vi "PortsArrayHandler.vi"(2 "Input":u8[](array[numeric]), 3 "Init Input":u8[](array[numeric]), 4 "INPUT PORT states":bool[](array[boolean])) -> (0 "Rezult Input Ports":u8[](array[numeric]))   [LabVIEW 2009]
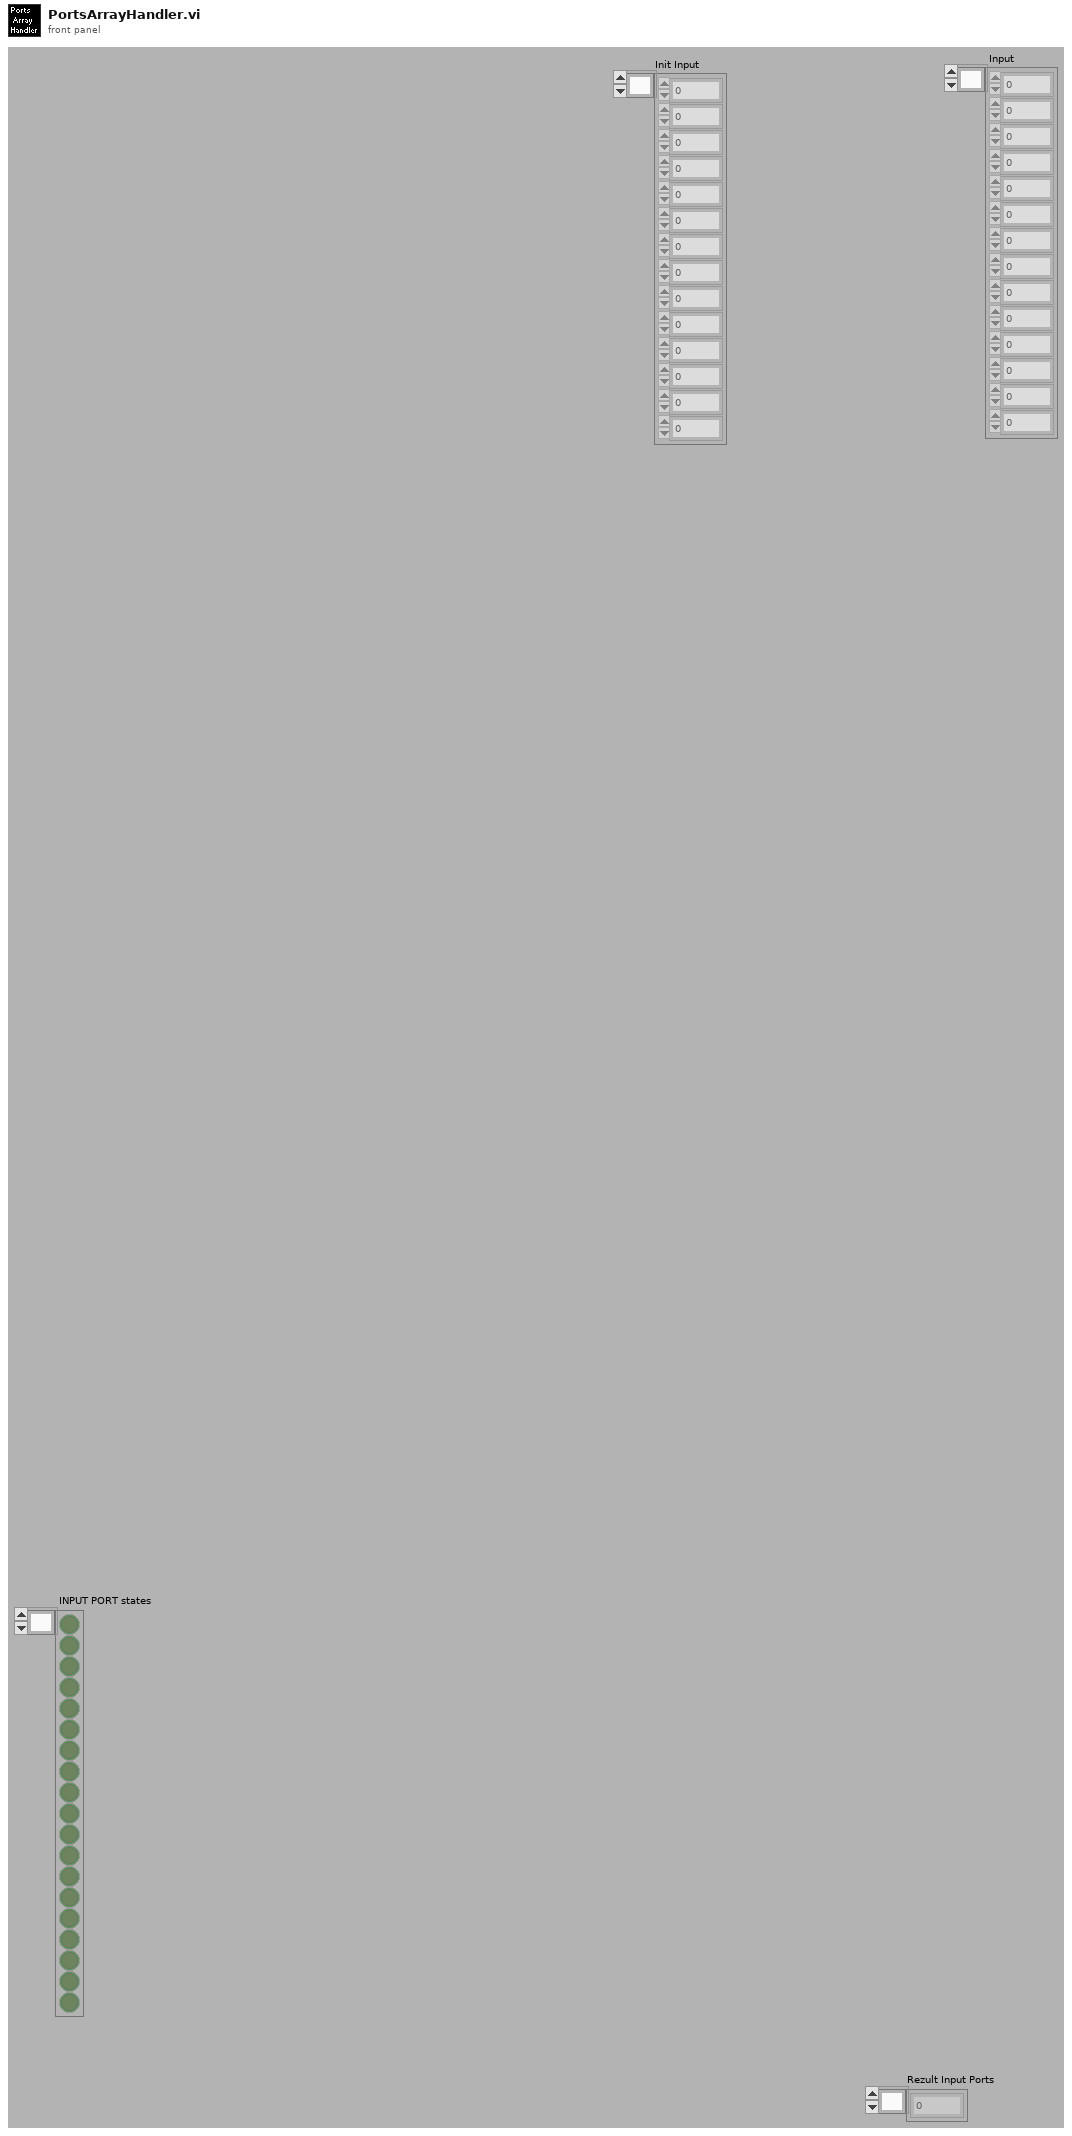
[diagram p1: front panel]
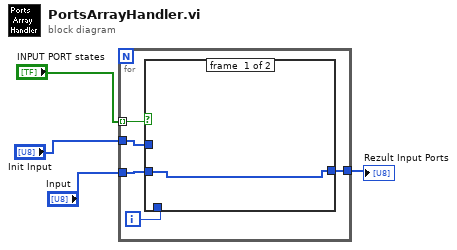
[diagram p0: block diagram]
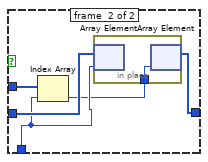
[diagram p2: hidden frame]
diagram:
  n1 = for {
    tunnel: "Input" -> [w8]
    tunnel: "INPUT PORT states" -> [w9] mode=indexing
    tunnel: "Init Input" -> [w6]
    tunnel: [w5] -> w1
    i -> [w7]
    n2 = case shown="True" w9 {
      tunnel: w8 -> [w10 w14]
      tunnel: w7 -> [_ w12]
      tunnel: w6 -> [_ w15]
      tunnel: [w10 w13] -> w5
      frame #0 {
      }
      frame #1 {
        n3 = Index Array(array=w15, index=w12) -> (element=w11:u8)
        n4 = in-place {
          in-place-border: w11 -> [w16]
          n5 = in-place-array #1(w14, w12) -> ()  [unwired: 1 out]
          n6 = in-place-array #1(w16) -> (w13:u8[])  [unwired: 1 out]
        }
      }
    }
  }
  "Rezult Input Ports" <- w1
